vi "LOG.vi"(8 "error in (no error)":errorcluster, 11 "Queues":T1) -> (0 "error out":errorcluster)   [LabVIEW 2014]
uses:
  CMD UI enum.ctl
  CMD Report enum.ctl
  CMD DA enum.ctl
  CMD DAQ enum.ctl
  CMD LOG enum.ctl
  set_get.ctl
  patiant and daq params.ctl
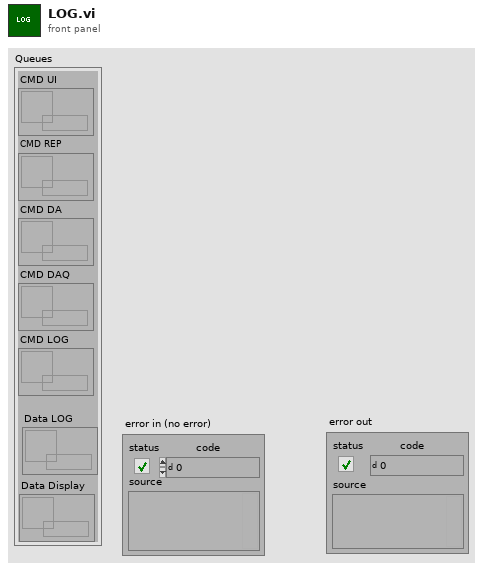
[diagram p1: front panel]
types:
  T1 = cluster{"CMD UI":refnum<queue>, "CMD REP":refnum<queue>, "CMD DA":refnum<queue>, "CMD DAQ":refnum<queue>, "CMD LOG":refnum<queue>, "Data LOG":refnum<queue>, "Data Display":refnum<queue>}
  T2 = typedef "patiant and daq params.ctl" = cluster{"DAQ Parameters":cluster{"Sampling rate":dbl, "Max_volt":dbl, "Min_volt":dbl, "DAQmx Physical Channels \nHR,SC":tag, "Resting State":bool, "Analyze every (s)":dbl}, "Patient Info \n(Updates automatically when reading from file)":cluster{"Patient Name":string, "Patient ID":string, "Patient Age":dbl, "Gender":string}, "Raw Data Read Path":path, "Avg HR ":dbl, "Avg SC  ":dbl}
  T3 = typedef "CMD LOG enum.ctl" = enum16{"Start Log", "Log", "Stop Log", "Exit"}
  T4 = typedef "set_get.ctl" = enum16{"Set", "Get"}
  T5 = enum16{"open", "replace", "create", "open or create", "replace or create", "replace or create with confirmation"}
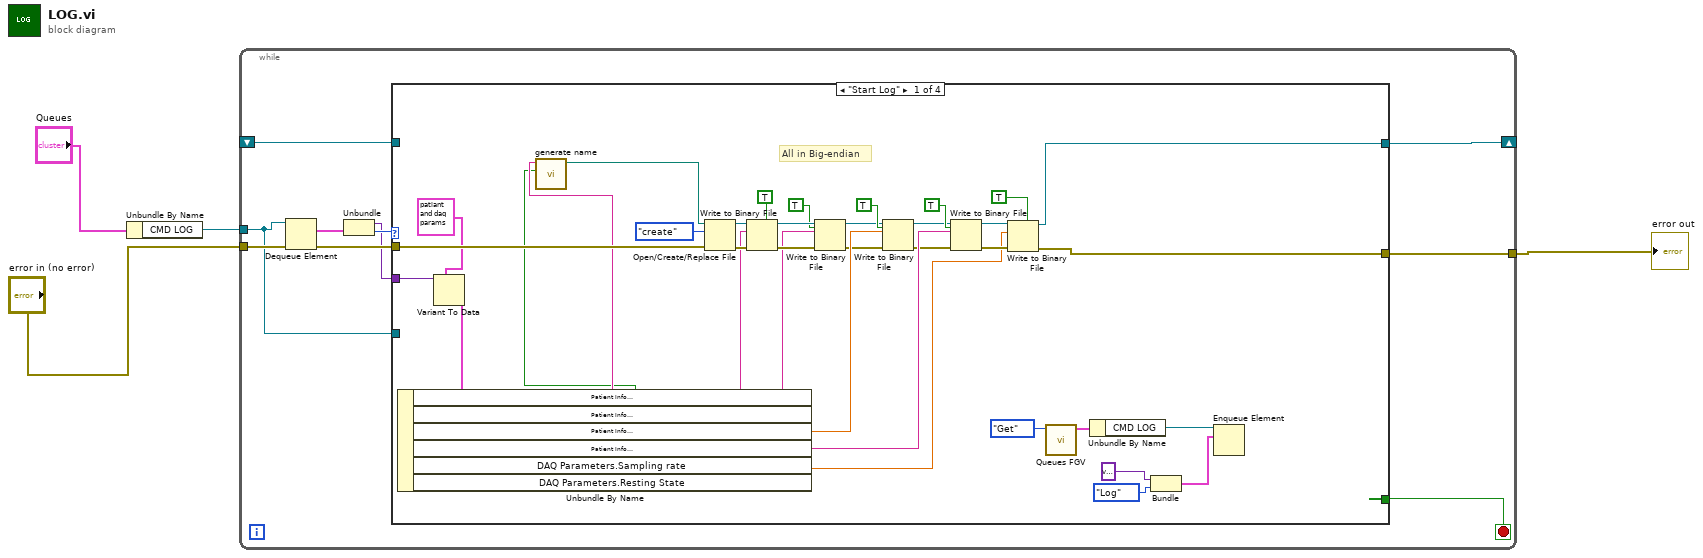
[diagram p0: block diagram]
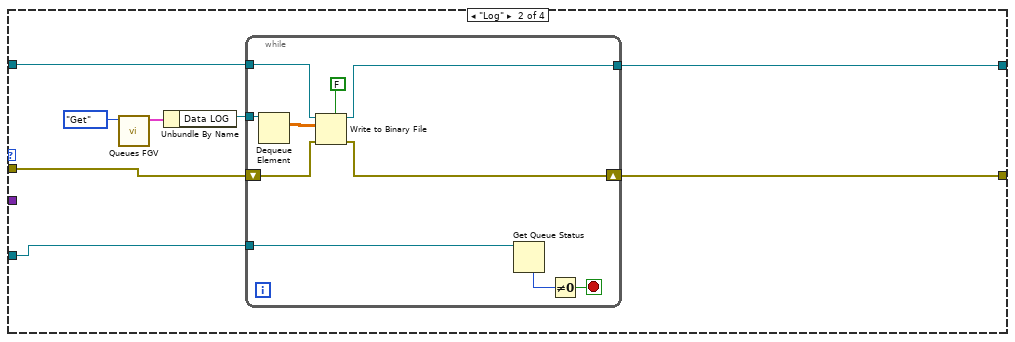
[diagram p2: hidden frame]
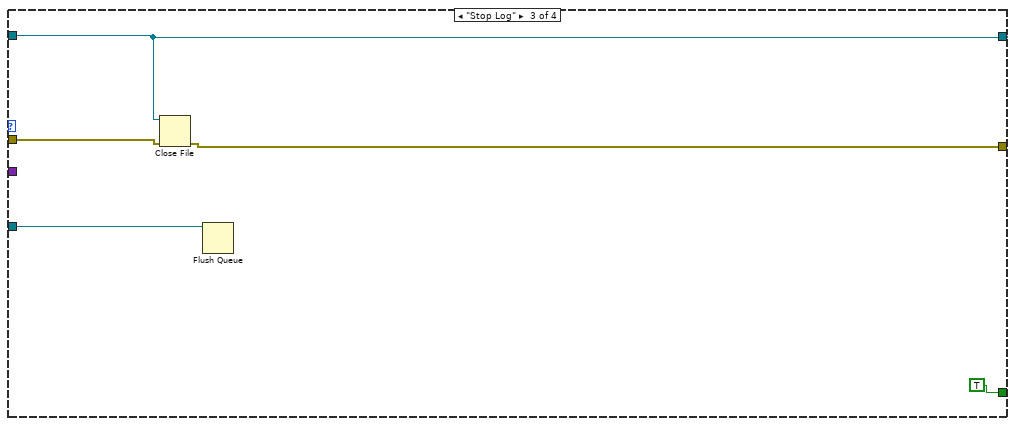
[diagram p3: hidden frame]
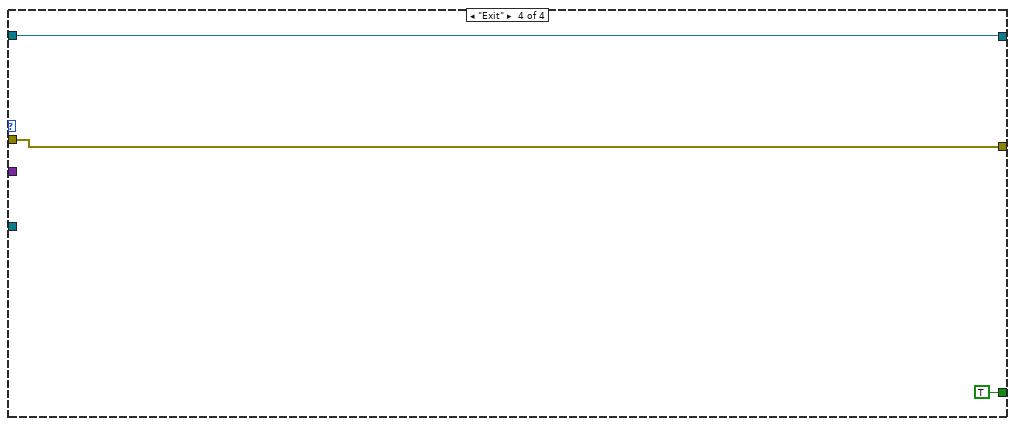
[diagram p4: hidden frame]
diagram:
  n1 = Unbundle By Name("Queues") -> ("CMD LOG"=w4:refnum<queue>)
  n2 = while {
    tunnel: w4 -> [w5]
    tunnel: [w11] -> w3
    shift-right: [w10] -> _
    shift-left: _ -> [w9]
    tunnel: "error in (no error)" -> [w7]
    stop <- w8 stop-if-true
    n3 = Dequeue Element(queue=w5, error in (no error)=w7) -> (element=w14:cluster{variant, T3}, error out=w12:errorcluster)  [unwired: 1 in, 2 out]
    n4 = Unbundle(w14) -> (w6:variant, w13:T3)
    n5 = case shown="\"Start Log\"" w13 {
      tunnel: w12 -> [w48 w53 w70 w74]
      tunnel: [w16 w52 w72 w74] -> w11
      tunnel: [w15 w51 w69 w75] -> w10
      tunnel: w9 -> [_ w57 w69 w75]
      tunnel: [_ _ TRUE TRUE] -> w8
      tunnel: w6 -> [w32 _ _ _]
      tunnel: w5 -> [_ w50 w68 _]
      frame "Start Log" {
        # "All in Big-endian"
        n6 = Variant To Data(type=T2 {"DAQ Parameters"={"Sampling rate"=0.0, "Max_volt"=1000.0, "Min_volt"=0.0, "DAQmx Physical Channels \nHR,SC"="", "Resting State"=FALSE, "Analyze every (s)"=0.01}, "Patient Info \n(Updates automatically when reading from file)"={"Patient Name"="", "Patient ID"="", "Patient Age"=0.0, "Gender"=""}, "Raw Data Read Path"=path "", "Avg HR "=0.0, "Avg SC  "=0.0} ("The Cluster"), Variant=w32) -> (data=w31:T2)  [unwired: 1 in, 1 out]
        n7 = Unbundle By Name(w31) -> ("Patient Info \n(Updates automatically when reading from file).Patient Name"=w19:string, "Patient Info \n(Updates automatically when reading from file).Patient ID"=w42:string, "Patient Info \n(Updates automatically when reading from file).Patient Age"=w39:dbl, "Patient Info \n(Updates automatically when reading from file).Gender"=w35:string, "DAQ Parameters.Sampling rate"=w22:dbl, "DAQ Parameters.Resting State"=w17:bool)
        n8 = call "generate name.vi"("rest (T) active (F)"=w17, "Patient Name"=w19) -> ("appended path"=w20:path)  [unwired: 9 in]
        n9 = Open/Create/Replace File(file path (use dialog)=w20, error in=w48, operation (0:open)=T5."create") -> (refnum out=w47:refnum<file>, error out=w46:errorcluster)  [unwired: 3 in, 1 out]
        n10 = Write to Binary File(file (use dialog)=w47, data=w19, error in=w46, 5:TRUE ("prepend array or string size? (T)")) -> (refnum out=w43:refnum<file>, error out=w44:errorcluster)  [unwired: 2 in, 1 out]
        n11 = Write to Binary File(file (use dialog)=w43, data=w42, error in=w44, 5:TRUE ("prepend array or string size? (T)")) -> (refnum out=w37:refnum<file>, error out=w38:errorcluster)  [unwired: 2 in, 1 out]
        n12 = Write to Binary File(file (use dialog)=w37, data=w39, error in=w38, 5:TRUE ("prepend array or string size? (T)")) -> (refnum out=w34:refnum<file>, error out=w33:errorcluster)  [unwired: 2 in, 1 out]
        n13 = Write to Binary File(file (use dialog)=w34, data=w35, error in=w33, 5:TRUE ("prepend array or string size? (T)")) -> (refnum out=w23:refnum<file>, error out=w24:errorcluster)  [unwired: 2 in, 1 out]
        n14 = Write to Binary File(file (use dialog)=w23, data=w22, error in=w24, 5:TRUE ("prepend array or string size? (T)")) -> (refnum out=w15:refnum<file>, error out=w16:errorcluster)  [unwired: 2 in, 1 out]
        n15 = call "Queues FGV.vi"("Enum"=set_get."Get") -> ("Queues"=w30:T1)  [unwired: 10 in]
        n16 = Unbundle By Name(w30) -> ("CMD LOG"=w28:refnum<queue>)
        n17 = Bundle(variant, "Enum"=CMD_LOG_enum."Log") -> (w25:cluster{variant, "Enum":T3})  [unwired: 1 in]
        n18 = Enqueue Element(queue=w28, element=w25) -> ()  [unwired: 2 in, 3 out]
      }
      frame "Log" {
        n19 = call "Queues FGV.vi"("Enum"=set_get."Get") -> ("Queues"=w56:T1)  [unwired: 10 in]
        n20 = Unbundle By Name(w56) -> ("Data LOG"=w54:refnum<queue>)
        n21 = while {
          tunnel: w57 -> [w67]
          tunnel: w54 -> [w66]
          tunnel: [w62] -> w51
          shift-right: [w63] -> w52
          shift-left: w53 -> [w64]
          tunnel: w50 -> [w59]
          stop <- w60 stop-if-true
          n22 = Dequeue Element(queue=w66) -> (element=w65:dbl[][])  [unwired: 2 in, 3 out]
          n23 = Write to Binary File(file (use dialog)=w67, data=w65, error in=w64, 5:FALSE ("prepend array or string size? (T)")) -> (refnum out=w62:refnum<file>, error out=w63:errorcluster)  [unwired: 2 in, 1 out]
          n24 = Get Queue Status(queue=w59) -> (# elements in queue=w61:i32)  [unwired: 2 in, 7 out]
          n25 = Not Equal To 0?(x=w61) -> (x != 0?=w60:bool)
        }
      }
      frame "Stop Log" {
        n26 = Close File(refnum=w69, error in=w70) -> (error out=w72:errorcluster)  [unwired: 1 out]
        n27 = Flush Queue(queue=w68) -> ()  [unwired: 1 in, 3 out]
      }
      frame "Exit" {
      }
    }
  }
  "error out" <- w3
